vi "GOOP_LVClass_Item_Interface.vi"() -> (3 "InterfaceTable":T1)   [LabVIEW 2016]
uses:
  <resource>/Framework/Providers/API/Item_Interface.ctl
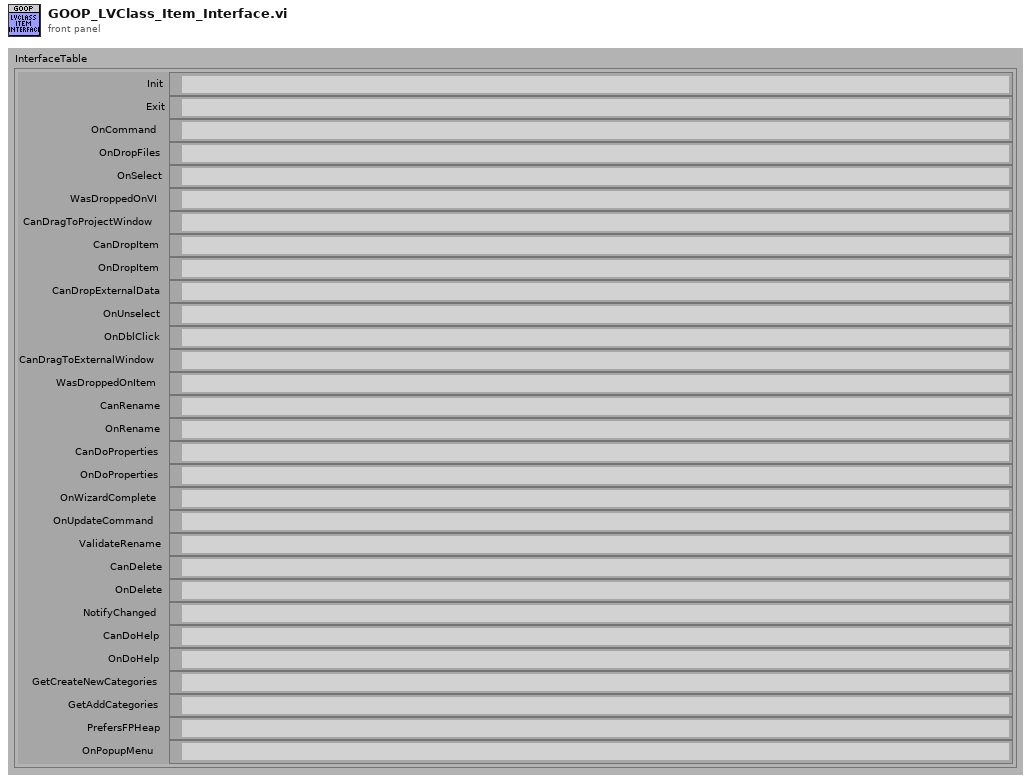
[diagram p1: front panel]
types:
  T1 = typedef "Item_Interface.ctl" = cluster{"Init":path, "Exit":path, "OnCommand":path, "OnDropFiles":path, "OnSelect":path, "WasDroppedOnVI":path, "CanDragToProjectWindow":path, "CanDropItem":path, "OnDropItem":path, "CanDropExternalData":path, "OnUnselect":path, "OnDblClick":path, "CanDragToExternalWindow":path, "WasDroppedOnItem":path, "CanRename":path, "OnRename":path, "CanDoProperties":path, "OnDoProperties":path, "OnWizardComplete":path, "OnUpdateCommand":path, "ValidateRename":path, "CanDelete":path, "OnDelete":path, "NotifyChanged":path, "CanDoHelp":path, "OnDoHelp":path, "GetCreateNewCategories":path, "GetAddCategories":path, "PrefersFPHeap":path, "OnPopupMenu":path}
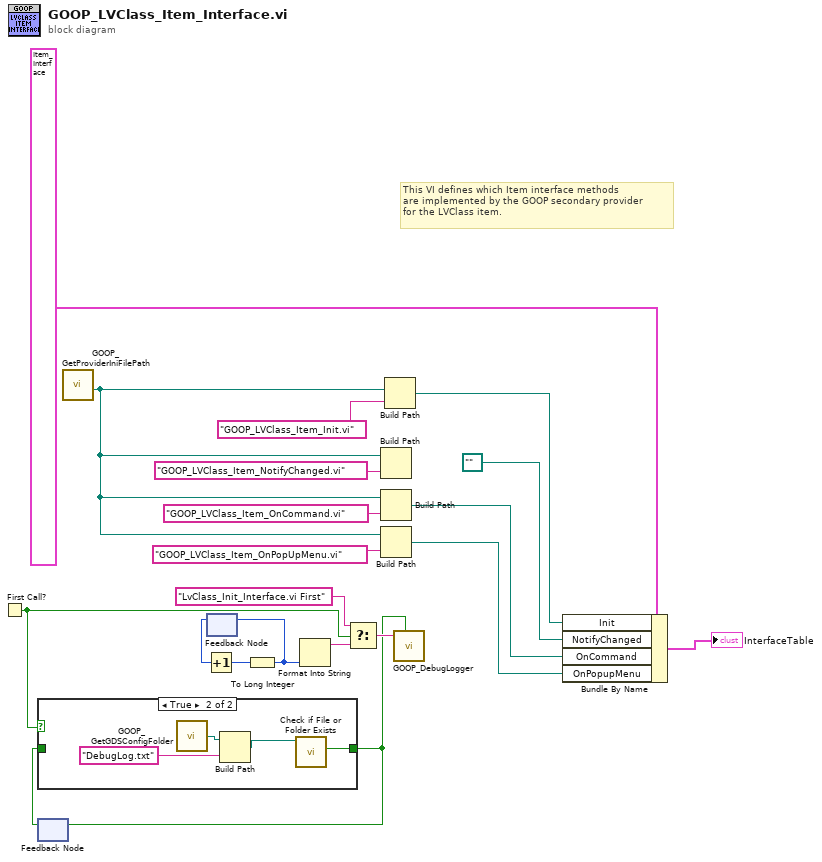
[diagram p0: block diagram]
diagram:
  # "This VI defines which Item interface methods \nare implemented by the GOOP secondary provider \nfor the LVClass item."
  n1 = First Call?() -> (First Call?: T/F=w2:bool)
  n2 = feedback #1() -> (w3:bool)  [unwired: 1 in]
  n3 = case shown="True" w2 {
    tunnel: [w21 w25] -> w1
    tunnel: w3 -> [w21 _]
    frame False {
    }
    frame True {
      n4 = call <resource>:"GOOP_GetGDSConfigFolder.vi"() -> ("GDSFolderPath"=w23:path)
      n5 = Build Path(base path=w23, name or relative path="DebugLog.txt") -> (appended path=w22:path)
      n6 = call <vilib>:"Check if File or Folder Exists.vi"("path"=w22) -> ("file or folder exists?"=w25:bool)  [unwired: 8 in, 2 out]
    }
  }
  n7 = feedback-in #1(w1) -> ()
  n8 = call <resource>:"GOOP_GetProviderIniFilePath.vi"() -> ("ProviderMainFolder"=w15:path)  [unwired: 10 in, 1 out]
  n9 = feedback #2() -> (w7:i32)  [unwired: 1 in]
  n10 = Increment(x=w7) -> (x+1=w6:i32)
  n11 = To Long Integer(number=w6) -> (32bit integer=w5:i32)
  n12 = feedback-in #2(w5) -> ()
  n13 = Format Into String(w5) -> (resulting string=w4:string)  [unwired: 3 in, 1 out]
  n14 = Select(t="LvClass_Init_Interface.vi First" ("name or relative path"), s=w2, f=w4) -> (s? t:f=w9:string)
  n15 = Build Path(base path=w15, name or relative path="GOOP_LVClass_Item_NotifyChanged.vi") -> ()  [unwired: 1 out]
  n16 = Build Path(base path=w15, name or relative path="GOOP_LVClass_Item_OnCommand.vi") -> (appended path=w11:path)
  n17 = Build Path(base path=w15, name or relative path="GOOP_LVClass_Item_OnPopUpMenu.vi") -> (appended path=w10:path)
  n18 = Build Path(base path=w15, name or relative path="GOOP_LVClass_Item_Init.vi") -> (appended path=w13:path)
  n19 = call <resource>:"GOOP_DebugLogger.vi"("ActivateDebugging"=w1, "State"=w9) -> ()  [unwired: 7 in, 3 out]
  n20 = Bundle By Name(cluster=T1 {"Init"=path "", "Exit"=path "", "OnCommand"=path "", "OnDropFiles"=path "", "OnSelect"=path "", "WasDroppedOnVI"=path "", "CanDragToProjectWindow"=path "", "CanDropItem"=path "", "OnDropItem"=path "", "CanDropExternalData"=path "", "OnUnselect"=path "", "OnDblClick"=path "", "CanDragToExternalWindow"=path "", "WasDroppedOnItem"=path "", "CanRename"=path "", "OnRename"=path "", "CanDoProperties"=path "", "OnDoProperties"=path "", "OnWizardComplete"=path "", "OnUpdateCommand"=path "", "ValidateRename"=path "", "CanDelete"=path "", "OnDelete"=path "", "NotifyChanged"=path "", "CanDoHelp"=path "", "OnDoHelp"=path "", "GetCreateNewCategories"=path "", "GetAddCategories"=path "", "PrefersFPHeap"=path "", "OnPopupMenu"=path ""} ("InterfaceTable"), "Init"=w13, "NotifyChanged"=path "", "OnCommand"=w11, "OnPopupMenu"=w10) -> (→"InterfaceTable":T1)
